vi "test Send from Nested and Stop.vi"(8 "error in (no error)":errorcluster, 11 "TestCase in":refnum<class "Test TCP Nested and Caller Endpoints.lvclass">) -> (0 "error out":errorcluster, 3 "TestCase out":refnum<class "Test TCP Nested and Caller Endpoints.lvclass">)   [LabVIEW 2020, in "Test TCP Nested and Caller Endpoints.lvclass"]
uses:
  Test TCP Nested and Caller Endpoints.lvclass
  <vilib>/addons/_JKI Toolkits/VI Tester/TestCase.llb/TestCase.lvclass
  <vilib>/ActorFramework/Message Queue/Message Queue.lvclass
  <vilib>/ActorFramework/LastAck/Last Ack.lvclass
  <vilib>/ActorFramework/Message Dequeuer/Message Dequeuer.lvclass
  Support/Caller Test Harness/Caller Test Harness Messages/Write String Data Msg/Write String Data Msg.lvclass
  Support/Caller Test Harness/Caller Test Harness/Caller Test Harness.lvclass
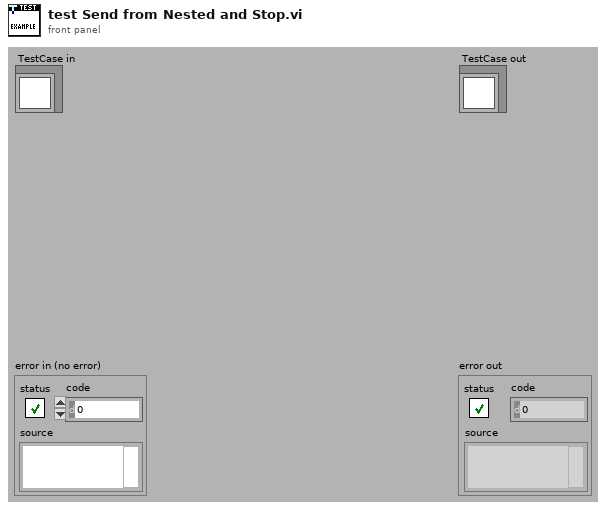
[diagram p1: front panel]
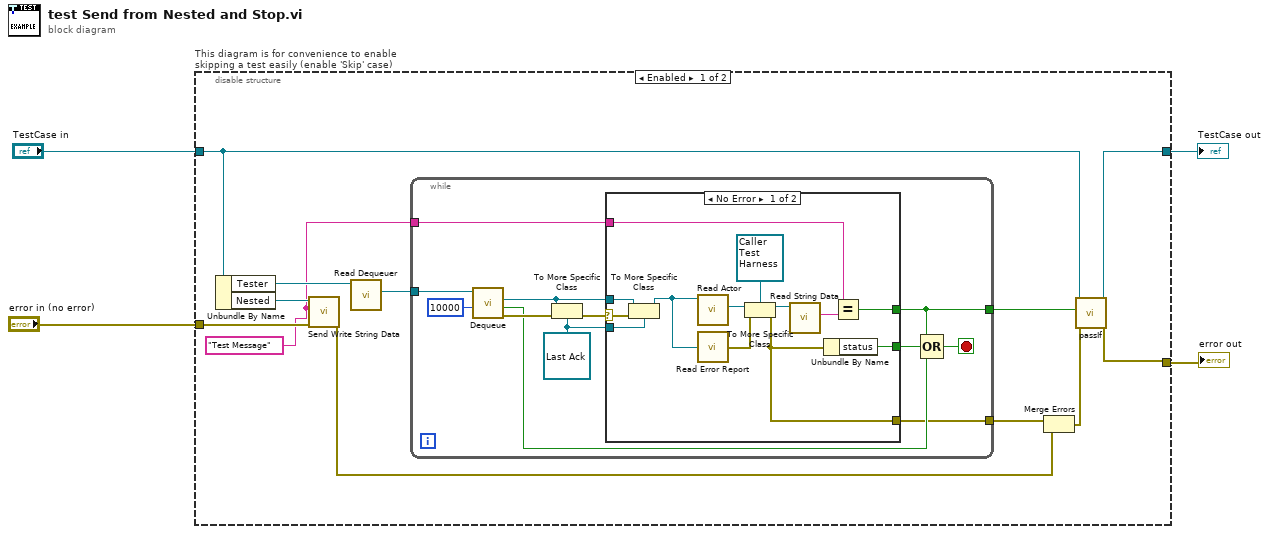
[diagram p0: block diagram]
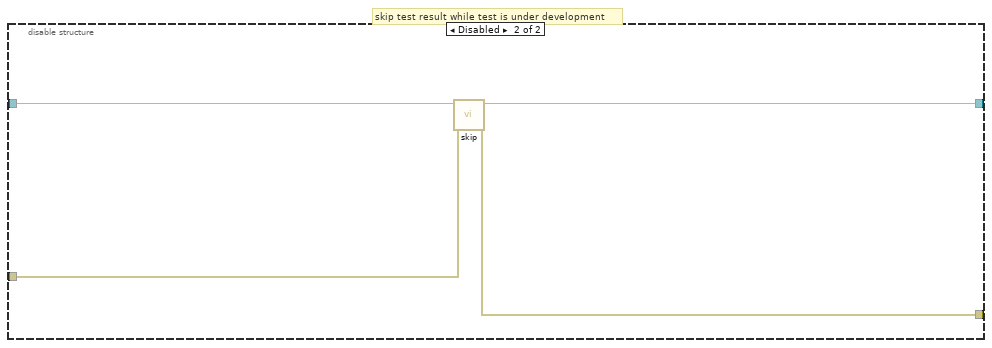
[diagram p3: hidden frame]
diagram:
  n1 = disable-structure "This diagram is for convenience to enable skipping a test easily (enable 'Skip' case)" shown="Enabled" {
    disable-tunnel: "TestCase in" -> [w14 w45]
    disable-tunnel: [w16 w43] -> w1
    disable-tunnel: [w15 w44] -> w3
    disable-tunnel: "error in (no error)" -> [w7 w42]
    frame Enabled {
      w5 = "Test Message" ("String Data")
      n2 = Unbundle By Name(w14) -> ("Tester"=w13:refnum<class "Message Queue.lvclass">, "Nested"=w8:refnum<class "Message Enqueuer.lvclass">)
      n3 = call "Send Write String Data.vi"("error in (no error)"=w7, "String Data"=w5, "Message Enqueuer"=w8) -> ("error out"=w6:errorcluster)  [unwired: 7 in, 1 out]
      n4 = call <vilib>:"Read Dequeuer.vi"("Message Queue"=w13) -> ("Message Dequeuer"=w11:refnum<class "Message Dequeuer.lvclass">)  [unwired: 10 in]
      n5 = while {
        tunnel: w11 -> [w28]
        tunnel: [w22] -> w10
        tunnel: [w21] -> w9
        tunnel: w5 -> [w17]
        stop <- w24 stop-if-true
        w18 = refnum<class "Last Ack.lvclass"> refnum ("Last Ack")
        n6 = call <vilib>:"Dequeue.vi"("timeout in ms (-1)"=10000, "Message Dequeuer in"=w28) -> ("error out"=w26:errorcluster, "timed out?"=w23:bool, "Message"=w19:refnum<class "Message.lvclass">)  [unwired: 5 in, 2 out]
        n7 = To More Specific Class(target class=w18, reference=w19, error in=w26) -> (error out=w20:errorcluster)  [unwired: 1 out]
        n8 = case shown="No Error" w20 {
          selector: w20 -> [w40 _]
          tunnel: [w41 _] -> w25
          tunnel: [w29 _] -> w22
          tunnel: [w34 _] -> w21
          tunnel: w19 -> [w39 _]
          tunnel: w18 -> [w38 _]
          tunnel: w17 -> [w30 _]
          frame No Error {
            n9 = To More Specific Class(target class=w38, reference=w39, error in=w40) -> (specific class reference=w37:refnum<class "Last Ack.lvclass">)  [unwired: 1 out]
            n10 = call <vilib>:"Read Actor.vi"("Last Ack"=w37) -> ("Actor"=w36:refnum<class "Actor.lvclass">)  [unwired: 10 in]
            n11 = call <vilib>:"Read Error Report.vi"("Last Ack"=w37) -> ("error report"=w33:errorcluster)
            n12 = To More Specific Class(target class=refnum<class "Caller Test Harness.lvclass"> refnum ("Caller Test Harness.lvlib:Caller Test Harness.lvclass"), reference=w36, error in=w33) -> (specific class reference=w32:refnum<class "Caller Test Harness.lvclass">, error out=w34:errorcluster)
            n13 = call "Read String Data.vi"("Caller Test Harness in"=w32) -> ("String Data"=w31:string)  [unwired: 10 in]
            n14 = Unbundle By Name(w34) -> ("status"=w41:bool)
            n15 = Equal?(x=w30, y=w31) -> (x = y?=w29:bool)
          }
          frame Error {
          }
        }
        n16 = Compound Arithmetic op=OR(w22, w25, w23) -> (w24:bool)
      }
      n17 = Merge Errors(w9, w6) -> (w12:errorcluster)
      n18 = call-dynamic "passIf.vi"("error in (no error)"=w12, "pass"=w10, "TestCase in"=w14) -> ("error out"=w15:errorcluster, "TestCase out"=w16:refnum<class "Test TCP Nested and Caller Endpoints.lvclass">)  [unwired: 7 in]
    }
    frame Disabled {
      # "skip test result while test is under development"
      n19 = call <vilib>:"skip.vi"("error in (no error)"=w42, "TestCase in"=w45) -> ("error out"=w44:errorcluster, "TestCase out"=w43:refnum<class "Test TCP Nested and Caller Endpoints.lvclass">)  [unwired: 8 in]
    }
  }
  "error out" <- w3
  "TestCase out" <- w1
